vi "Feed Forward Shooter Ramp.vi"(10 "Current RPM":dbl, 11 "Target RPM":dbl) -> (3 "Ramped Output":dbl)   [LabVIEW 2015]
uses:
  Common Code/Change Detect Boolean.vi
  Robot Code/Robot Global Data.vi
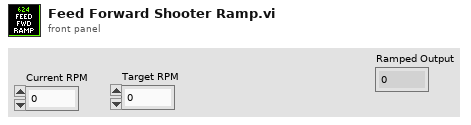
[diagram p1: front panel]
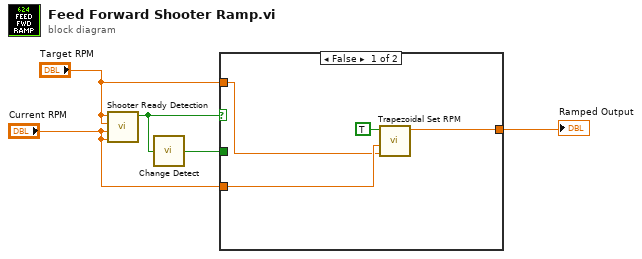
[diagram p0: block diagram]
diagram:
  n1 = call "Shooter Ready Detection.vi"("Right RPM"="Current RPM", "Left RPM"="Current RPM", "Right RPM Target"="Target RPM", "Left RPM Target"="Target RPM") -> ("Shooter Ready?"=w3:bool)  [unwired: 7 in]
  n2 = call-poly "Change Detect.vi"("In"=w3) -> ("Changed?"=w2:bool)
  n3 = case shown="False" w3 {
    tunnel: "Target RPM" -> [w7 w10]
    tunnel: [w6 w10] -> w4
    tunnel: w2 -> [_ _]
    tunnel: "Current RPM" -> [w8 _]
    frame False {
      n4 = call "Trapezoidal Set RPM.vi"("Desired RPM"=w7, "Current RPM"=w8, "Spinning Wheels?"=TRUE) -> ("RPM"=w6:dbl)  [unwired: 6 in, 2 out]
    }
    frame True {
    }
  }
  "Ramped Output" <- w4
